vi "set trigger.vi"(8 "error in (no error)":errorcluster, 11 "Thorcam in":refnum<class "Thorcam.lvclass">) -> (0 "error out":errorcluster, 3 "Thorcam out":refnum<class "Thorcam.lvclass">)   [LabVIEW 2012]
uses:
  Thorcam.lvclass
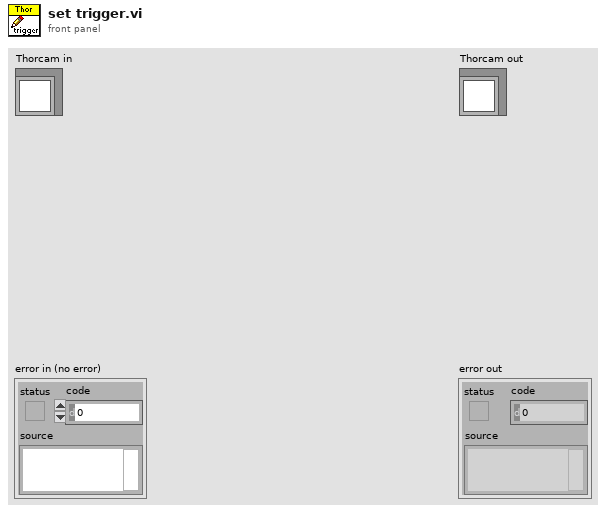
[diagram p1: front panel]
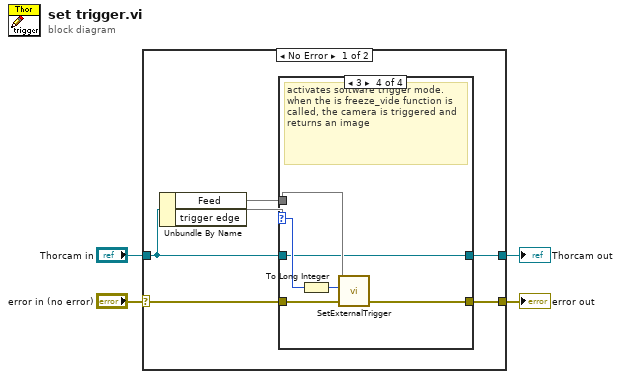
[diagram p0: block diagram]
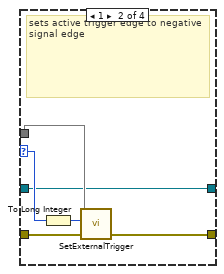
[diagram p3: hidden frame]
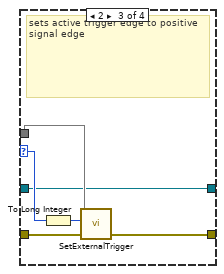
[diagram p4: hidden frame]
diagram:
  n1 = case shown="No Error" "error in (no error)" {
    selector: "error in (no error)" -> [w9 w32]
    tunnel: [w8 w32] -> w3
    tunnel: [w6 w31] -> w1
    tunnel: "Thorcam in" -> [w7 w31]
    frame No Error {
      n2 = Unbundle By Name(w7) -> ("Feed"=w10, "trigger edge"=w5)
      n3 = case shown="3" w5 {
        selector: w5 -> [_ w15 w21 w27]
        tunnel: w10 -> [_ w18 w24 w30]
        tunnel: w9 -> [w11 w17 w23 w29]
        tunnel: [w11 w16 w22 w28] -> w8
        tunnel: w7 -> [w12 w13 w19 w25]
        tunnel: [w12 w13 w19 w25] -> w6
        frame 0, Default {
          # "deactivates trigger processing"
        }
        frame 1 {
          # "sets active trigger edge to negative signal edge"
          n4 = To Long Integer(number=w15) -> (32bit integer=w14:i32)
          n5 = call <instrlib>:"SetExternalTrigger.vi"("error in"=w17, "Trigger Mode"=w14, "Camera Handle In"=w18) -> ("error out"=w16:errorcluster)  [unwired: 6 in, 2 out]
        }
        frame 2 {
          # "sets active trigger edge to positive signal edge"
          n6 = To Long Integer(number=w21) -> (32bit integer=w20:i32)
          n7 = call <instrlib>:"SetExternalTrigger.vi"("error in"=w23, "Trigger Mode"=w20, "Camera Handle In"=w24) -> ("error out"=w22:errorcluster)  [unwired: 6 in, 2 out]
        }
        frame 3 {
          # "activates software trigger mode. when the is freeze_vide function is called, the camera is triggered and returns an image"
          n8 = To Long Integer(number=w27) -> (32bit integer=w26:i32)
          n9 = call <instrlib>:"SetExternalTrigger.vi"("error in"=w29, "Trigger Mode"=w26, "Camera Handle In"=w30) -> ("error out"=w28:errorcluster)  [unwired: 6 in, 2 out]
        }
      }
    }
    frame Error {
    }
  }
  "error out" <- w3
  "Thorcam out" <- w1
